vi "galvoWriteWrite.vi"(0 "X":dbl, 1 "Y":dbl, 2 "write X (T)":bool=TRUE, 3 "write Y (T)":bool=TRUE, 4 "fractional units (T)":bool=TRUE) -> ()   [LabVIEW 2017]
uses:
  <vilib>/DAQmx/write.llb/DAQmx Write (Analog DBL 1Chan 1Samp).vi
  globalDevices.vi
  <vilib>/DAQmx/miscellaneous.llb/DAQmx Fill In Error Info.vi
panel:
  # "Input values in Volts or in fractional units"
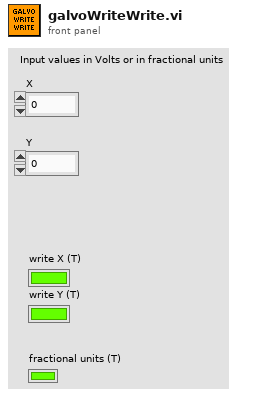
[diagram p1: front panel]
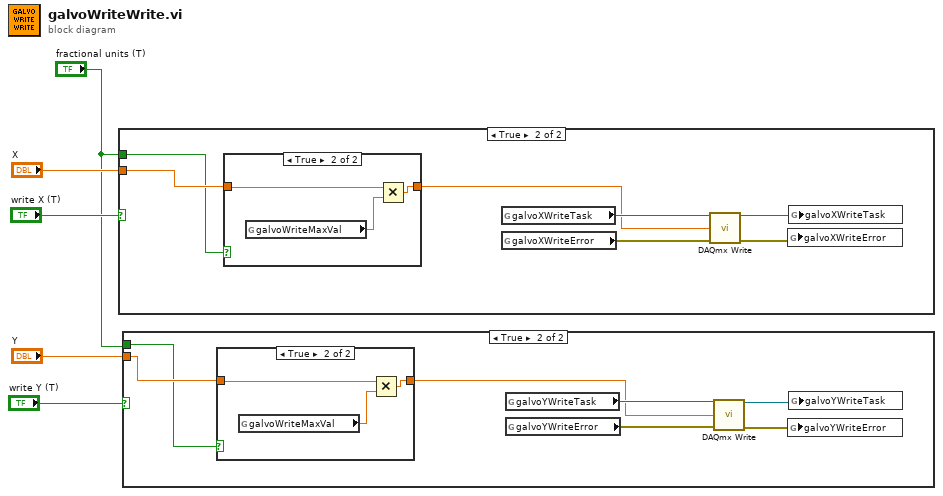
[diagram p0: block diagram]
diagram:
  n1 = case shown="True" "write X (T)" {
    tunnel: "X" -> [_ w8]
    tunnel: "fractional units (T)" -> [_ w6]
    frame False {
    }
    frame True {
      n2 = case shown="True" w6 {
        tunnel: w8 -> [w13 w16]
        tunnel: [w13 w14] -> w7
        frame False {
        }
        frame True {
          n3 = global read "globalDevices.vi" "galvoWriteMaxVal"() -> (w15:dbl)
          n4 = Multiply(x=w16, y=w15) -> (x*y=w14:dbl)
        }
      }
      n5 = global read "globalDevices.vi" "galvoXWriteTask"() -> (w12:refnum<k21>)
      n6 = global read "globalDevices.vi" "galvoXWriteError"() -> (w11:errorcluster)
      n7 = call-poly <vilib>:"DAQmx Write.vi"("task/channels in"=w12, "data"=w7, "error in"=w11) -> ("task out"=w10:refnum<k21>, "error out"=w9:errorcluster)  [unwired: 10 in, 1 out]
      n8 = global write "globalDevices.vi" "galvoXWriteError"(w9) -> ()
      n9 = global write "globalDevices.vi" "galvoXWriteTask"(w10) -> ()
    }
  }
  n10 = case shown="True" "write Y (T)" {
    tunnel: "Y" -> [_ w19]
    tunnel: "fractional units (T)" -> [_ w18]
    frame False {
    }
    frame True {
      n11 = case shown="True" w18 {
        tunnel: w19 -> [w24 w27]
        tunnel: [w24 w25] -> w17
        frame False {
        }
        frame True {
          n12 = global read "globalDevices.vi" "galvoWriteMaxVal"() -> (w26:dbl)
          n13 = Multiply(x=w27, y=w26) -> (x*y=w25:dbl)
        }
      }
      n14 = global read "globalDevices.vi" "galvoYWriteTask"() -> (w23:refnum<k21>)
      n15 = global read "globalDevices.vi" "galvoYWriteError"() -> (w22:errorcluster)
      n16 = call-poly <vilib>:"DAQmx Write.vi"("task/channels in"=w23, "data"=w17, "error in"=w22) -> ("task out"=w21:refnum<k21>, "error out"=w20:errorcluster)  [unwired: 10 in, 1 out]
      n17 = global write "globalDevices.vi" "galvoYWriteError"(w20) -> ()
      n18 = global write "globalDevices.vi" "galvoYWriteTask"(w21) -> ()
    }
  }
